vi "MAIN_display_new_image.vi"(4 "ROI":T1, 5 "Real time image":T2, 6 "error in":errorcluster, 7 "ROI Image":T2, 8 "Contrast image":T2, 9 "Image contrast":cluster{i32, i32}(slide)={16000, 0} scale=0.0..16000.0) -> (0 "error out":errorcluster, 1 "ROI":T2, 2 "Image":T2, 3 "Intensity range":cluster{sgl, sgl}(slide) scale=0.0..16000.0)   [LabVIEW 2015]
uses:
  <vilib>/vision/Image Controls.llb/IMAQ Image.ctl
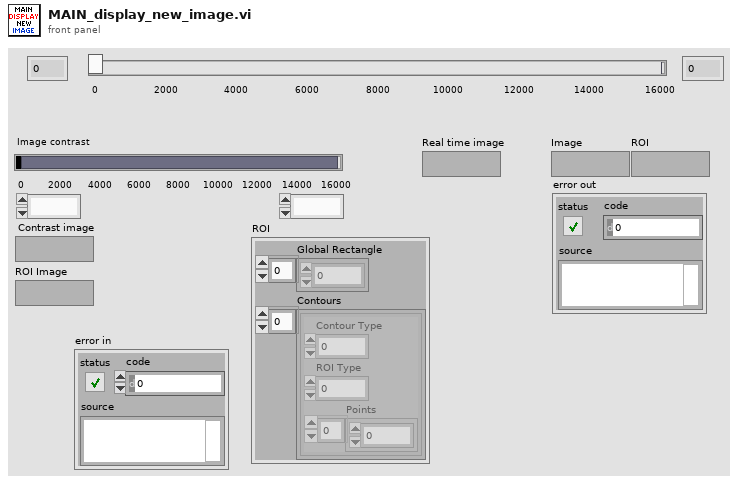
[diagram p1: front panel]
types:
  T1 = cluster{"Global Rectangle":i32[], "Contours":cluster{"Contour Type":u32, "ROI Type":u32, "Points":i32[]}[]}
  T2 = typedef "IMAQ Image.ctl" = refnum<image>
  T3 = cluster{"Maximal Value":sgl, "Minimal Value":sgl}
  T4 = cluster{"Mean Value":sgl, "Standard Variation":sgl, "Minimal Value":sgl, "Maximal Value":sgl, "Area (calibrated)":sgl, "Area (pixels)":u32, "%":sgl, "Calibration Valid":bool}
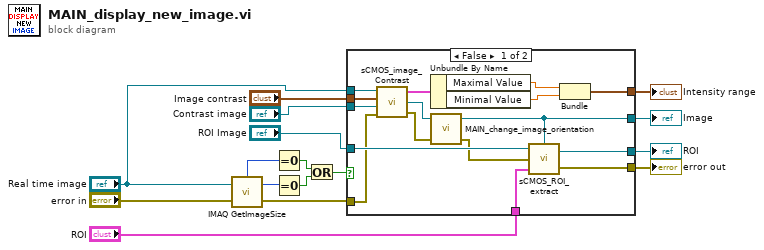
[diagram p0: block diagram]
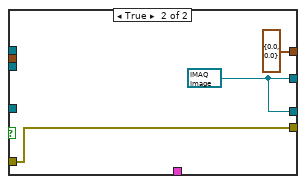
[diagram p2: hidden frame]
diagram:
  n1 = call "IMAQ GetImageSize"("Image"="Real time image", "error in (no error)"="error in") -> ("Y Resolution"=w14:i32, "X Resolution"=w13:i32, "error out"=w11:errorcluster)  [unwired: 2 in]
  n2 = Equal To 0?(x=w13) -> (x = 0?=w15:bool)
  n3 = Equal To 0?(x=w14) -> (x = 0?=w16:bool)
  n4 = Or(x=w15, y=w16) -> (x .or. y?=w10:bool)
  n5 = case shown="False" w10 {
    tunnel: "Contrast image" -> [w29 _]
    tunnel: "Image contrast" -> [w28 _]
    tunnel: "ROI Image" -> [w27 _]
    tunnel: [w26 w35] -> w1
    tunnel: w11 -> [w25 w35]
    tunnel: "Real time image" -> [w22 _]
    tunnel: [w21 T3 {"Maximal Value"=0.0, "Minimal Value"=0.0}] -> w5
    tunnel: [w20 w33] -> w4
    tunnel: [w18 w33] -> w3
    tunnel: "ROI" -> [w17 _]
    frame False {
      n6 = call "sCMOS_image_Contrast.vi"("error in"=w25, "Image Dst"=w29, "Image contrast"=w28, "New Image"=w22) -> ("error out"=w24:errorcluster, "Image Dst Out"=w23:T2, "Global Report"=w32:T4)
      n7 = Unbundle By Name(w32) -> ("Maximal Value"=w31:sgl, "Minimal Value"=w30:sgl)
      n8 = call "MAIN_change_image_orientation.vi"("error in"=w24, "Image IN"=w23) -> ("error out"=w19:errorcluster, "Image Out"=w20:T2)  [unwired: 2 in]
      n9 = call "sCMOS_ROI_extract.vi"("Image IN"=w20, "ROI"=w17, "error in"=w19, "Image ROI"=w27) -> ("error out"=w26:errorcluster, "Image Out"=w18:T2)
      n10 = Bundle("Maximal Value"=w31, "Minimal Value"=w30) -> (w21:T3)  [unwired: 1 in]
    }
    frame True {
      w33 = T2 refnum ("Image Out")
    }
  }
  "Intensity range" <- w5
  "Image" <- w4
  "ROI" <- w3
  "error out" <- w1
